vi "CHARGER_MICS, Telem Setup.vi"(6 "2.45 GHz Wake-Up Power (16)":i8(ring)=16 items=["-29"=-29, "-4"=-4, "-2"=-2, "0"=0, "2"=2, "4"=4, "6"=6, "8"=8, "10"=10, "12"=12, "14"=14, "16"=16, "18"=18, "20"=20, "22"=22, "24"=24, "26"=26, "27"=27], 8 "error in":errorcluster, 9 "Attenuation dB (25)":dbl=22.0, 10 "400 MHz MICS Power Setting (0x16)":u8=22 format="%02x", 11 "VISA resource":refnum<visa-resource-name>) -> (0 "error out":errorcluster, 3 "VISA resource dup":refnum<visa-resource-name>)   [LabVIEW 2020]
uses:
  Drivers/Telemetry/MICS Parameters Global.vi
  Drivers/Telemetry/MICS_ID Global.vi
  Drivers/Telemetry/MICS_Channel Global.vi
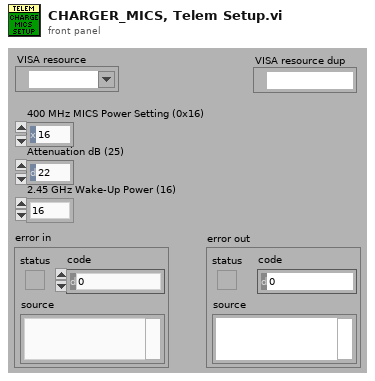
[diagram p1: front panel]
types:
  T1 = cluster{"ConfigFlags":u8, "ImplantID":u32, "CompanyID":u8, "Normal_Comm":cluster{"RF_Channel":u8, "UserData":u8, "TX_Mod":u8, "RX_Mod":u8, "RX_BlockSize":u8, "BlockPerPack":u8, "TX_BlockSize":u8}, "Emerg_Comm":cluster{"RF_Channel":u8, "UserData":u8, "TX_Mod":u8, "RX_Mod":u8, "TX_BlockSize":u8, "BlockPerPack":u8, "RX_BlockSize":u8}, "ImplantRev":u8, "245TX_PowerCal":i8, "245TX_Power":i8, "CCA_RSSI_Thresholds":cluster{"ch0":u16, "ch1":u16, "ch2":u16, "ch3":u16, "ch4":u16, "ch5":u16, "ch6":u16, "ch7":u16, "ch8":u16, "ch9":u16}}
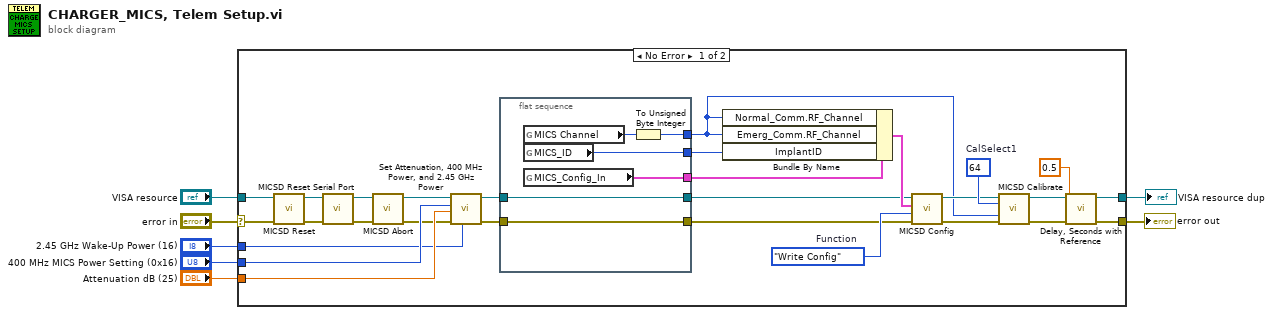
[diagram p0: block diagram]
diagram:
  n1 = case shown="No Error" "error in" {
    selector: "error in" -> [w30 w43]
    tunnel: "400 MHz MICS Power Setting (0x16)" -> [w22 _]
    tunnel: [w19 w43] -> w6
    tunnel: "VISA resource" -> [w31 w42]
    tunnel: "Attenuation dB (25)" -> [w23 _]
    tunnel: "2.45 GHz Wake-Up Power (16)" -> [w21 _]
    tunnel: [w20 w42] -> w1
    frame No Error {
      w29 = u8 64  # CalSelect1
      w28 = enum16{"Write Config", "Read Config"}."Write Config"  # Function
      n2 = call "MICSD Reset.vi"("error in (no error)"=w30, "VISA Resource Name"=w31) -> ("error out"=w35:errorcluster, "dup VISA Resource Name"=w34:refnum<visa-resource-name>)  [unwired: 8 in]
      n3 = call "MICSD Reset Serial Port.vi"("error in (no error)"=w35, "VISA Resource Name"=w34) -> ("error out"=w33:errorcluster, "dup VISA Resource Name"=w32:refnum<visa-resource-name>)  [unwired: 8 in]
      n4 = call "MICSD Abort.vi"("error in (no error)"=w33, "VISA Resource Name"=w32) -> ("error out"=w17:errorcluster, "dup VISA Resource Name"=w18:refnum<visa-resource-name>)  [unwired: 8 in]
      n5 = call "Set Attenuation, 400 MHz Power, and 2.45 GHz Power.vi"("2.45 GHz Wake-Up Power (6)"=w21, "error in"=w17, "Attenuation dB (0)"=w23, "400 MHz MICS Power Setting (0x16)"=w22, "VISA Resource Name"=w18) -> ("error out"=w12:errorcluster, "dup VISA Resource Name"=w14:refnum<visa-resource-name>)  [unwired: 5 in]
      n6 = flat-sequence {
        tunnel: w14 -> [w41]
        tunnel: [w41] -> w13
        tunnel: w12 -> [w40]
        tunnel: [w40] -> w11
        tunnel: [w39] -> w10
        tunnel: [w37] -> w9
        tunnel: [w36] -> w8
        frame #0 {
          n7 = global read "MICS_Channel Global.vi" "MICS Channel"() -> (w38:u16)
          n8 = global read "MICS_ID Global.vi" "MICS_ID"() -> (w36:u32)
          n9 = global read "MICS Parameters Global.vi" "MICS_Config_In"() -> (w39:T1)
          n10 = To Unsigned Byte Integer(number=w38) -> (unsigned 8bit integer=w37:u8)
        }
      }
      n11 = Bundle By Name(cluster=w10, "Normal_Comm.RF_Channel"=w9, "Emerg_Comm.RF_Channel"=w9, "ImplantID"=w8) -> (w27:T1)
      n12 = call "MICSD Config.vi"("error in (no error)"=w11, "Function"=w28, "MICS_Config_In"=w27, "VISA Resource Name"=w13) -> ("error out"=w15:errorcluster, "dup VISA Resource Name"=w16:refnum<visa-resource-name>)  [unwired: 5 in, 1 out]
      n13 = call "MICSD Calibrate.vi"("VISA Resource Name"=w16, "CalSelect1"=w29, "Channel"=w9, "error in (no error)"=w15) -> ("dup VISA Resource Name"=w24:refnum<visa-resource-name>, "error out"=w26:errorcluster)  [unwired: 10 in]
      n14 = call "Delay, Seconds with Reference.vi"("error in"=w26, "delay"=dbl[unit] 0.5, "VISA resource"=w24) -> ("error out"=w19:errorcluster, "VISA resource dup"=w20:refnum<visa-resource-name>)  [unwired: 3 in, 1 out]
    }
    frame Error {
    }
  }
  "error out" <- w6
  "VISA resource dup" <- w1
